vi "SLL Easy API Client Write Read Example.vi"() -> ()   [LabVIEW 2016, in "SLL Easy API via TCP.lvclass"]
doc: "SLL Easy API Client Write Read Example. \n\nRun the Server example before running this Client Example."
uses:
  SLL Easy API via TCP.lvclass
  _SubVIs/TCP Initialize Client - Local.vi
panel:
  out "error out":errorcluster
  out "Read Data":string
  in  "Write Data":string="Send Data and Receive Response"
  in  "Service Name":string="SLL Easy TCP Service"
  # "Run the Server VI Example before running this VI"
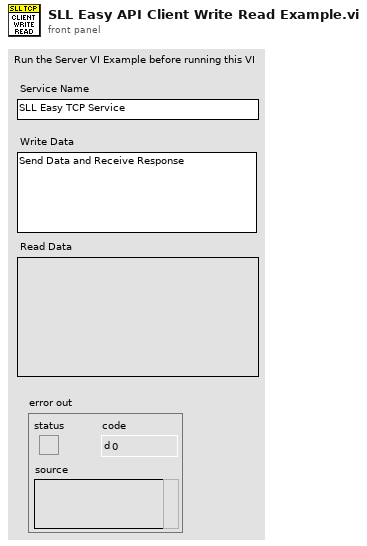
[diagram p1: front panel]
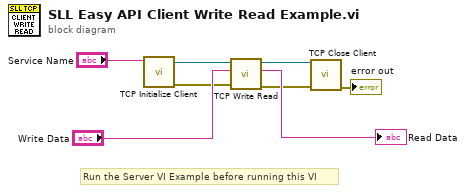
[diagram p0: block diagram]
diagram:
  # "Run the Server VI Example before running this VI"
  n1 = call-poly "TCP Initialize Client.vi"("Service Name"="Service Name") -> ("error out"=w4:errorcluster, "connection ID Out"=w8:refnum<k5>)  [unwired: 9 in]
  n2 = call "TCP Write Read.vi"("error in (no error)"=w4, "Write Data"="Write Data", "connection ID In"=w8) -> ("error out"=w3:errorcluster, "Read Data"=→"Read Data":string, "connection ID Out"=w7:refnum<k5>)  [unwired: 5 in, 1 out]
  n3 = call "TCP Close Client.vi"("error in (no error)"=w3, "connection ID"=w7) -> ("error out"=→"error out":errorcluster)  [unwired: 9 in]
